vi "PH_IEEE1394Camera.get further Cam Information.vi"(0 "i ref in":refnum<vi>, 2 "IMAQ1394 Session In":T1, 4 "Cam Error in":errorcluster, 5 "error in (no error)":errorcluster) -> (14 "i ref out":refnum<vi>, 16 "IMAQ1394 Session Out":T1, 18 "Cam Error out":errorcluster, 19 "error out":errorcluster)   [LabVIEW 2014, in "PH_IEEE1394Camera.lvlib"]
doc: "This VI gets the cam model and wrties it to own attributes and GUI element."
uses:
  PH_IEEE1394Camera.lvlib
  <vilib>/userdefined/High Color/IMAQdx.ctl
  <resource>/objmgr/imaqdx.rc
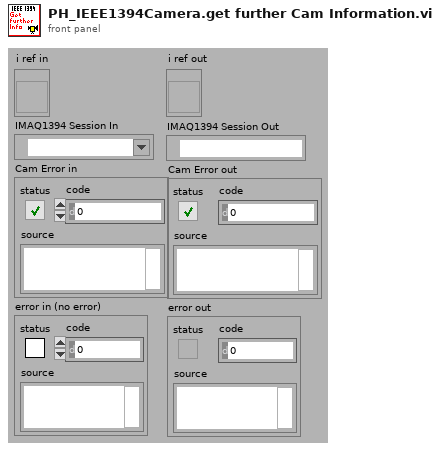
[diagram p1: front panel]
types:
  T1 = typedef "IMAQdx.ctl" = refnum<k21>
  T2 = typedef "PH_IEEE1394Camera.lvlib/PH_IEEE1394Camera.i attribute.ctl" = cluster{"Gui Refs":cluster{"Brightness":refnum<vi>, "Shutter":refnum<vi>, "Gain":refnum<vi>, "Center of Gravity":refnum<vi>, "Supported Video Modes":refnum<vi>, "Trigger Polarity":refnum<vi>, "Trigger Mode":refnum<vi>, "Trigger Timeout":refnum<vi>, "Bit Depth":refnum<vi>, "Video Mode":refnum<vi>, "Top":refnum<vi>, "Bottom":refnum<vi>, "Left":refnum<vi>, "Right":refnum<vi>, "Set ROI to Maximum":refnum<vi>, "Camera Details":refnum<vi>, "Current Cam Attributes":refnum<vi>, "Attribute to set":refnum<vi>, "Num Value":refnum<vi>, "String Value":refnum<vi>, "Bool Value":refnum<vi>, "Set Cam Attribute":refnum<vi>}, "Cam":cluster{"IMAQ1394 Session":T1, "Camera Details":T3}, "Current Attributes":T4[], "Supported Video Modes ":cluster{"Video Mode":u32, "Video Mode Name":string}[], "Wanted Attributes":cluster{"Name":string, "Num Value":dbl, "String Value":string, "Boolean Value":bool}[], "Cam Attributes":T6}
  T3 = typedef "PH_IEEE1394Camera.lvlib/PH_IEEE1394Camera.Cam Details.ctl" = cluster{"Model":string, "Serial Number":dbl, "Cam name (Machinery)":string, "Bus Type":string}
  T4 = typedef "PH_IEEE1394Camera.lvlib/PH_IEEE1394Camera.Cam Attribute.ctl" = cluster{"Information":cluster{"Type":T5, "Readable":bool, "Writable":bool, "Name":string}, "Num Value":dbl, "String Value":string, "Maximum":dbl, "Minimum":dbl, "Units":string, "Description":string, "EnumStrings[]":string[], "EnumValues[]":u32[], "Boolean Value":bool}
  T5 = typedef "NI_Vision_Acquisition_Software.lvlib/IMAQdx Attribute Type.ctl" = enum32{"U32", "I64", "DBL", "String", "Enum", "Bool", "Command"}
  T6 = typedef "PH_IEEE1394Camera.lvlib/PH_IEEE1394Camera.Relevant Cam Attributes.ctl" = cluster{"Video Mode":cluster{"Name":string, "Index":i32}, "Brightness":cluster{"Name":string, "Index":i32}, "Gain":cluster{"Name":string, "Index":i32}, "Shutter":cluster{"Name":string, "Index":i32}, "Trigger Pol":cluster{"Name":string, "Index":i32}, "Trigger Mode":cluster{"Name":string, "Index":i32}, "Timeout":cluster{"Name":string, "Index":i32}, "Bit Depth":cluster{"Name":string, "Index":i32}, "Pixel Bits":cluster{"Name":string, "Index":i32}, "Pixel Bytes":cluster{"Name":string, "Index":i32}, "Left":cluster{"Name":string, "Index":i32}, "Right":cluster{"Name":string, "Index":i32}, "Top":cluster{"Name":string, "Index":i32}, "Bottom":cluster{"Name":string, "Index":i32}}
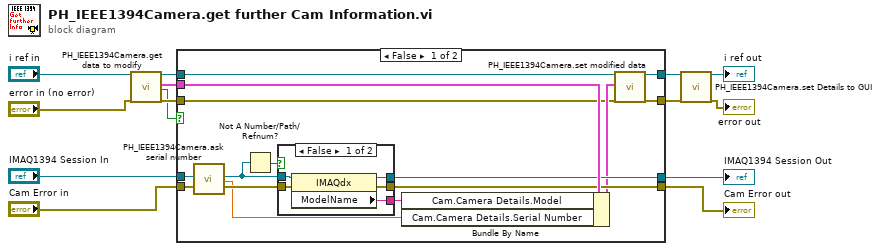
[diagram p0: block diagram]
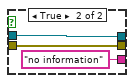
[diagram p2: hidden frame]
diagram:
  n1 = call "PH_IEEE1394Camera.get data to modify.vi"("i ref in"="i ref in", "error in (no error)"="error in (no error)") -> ("i ref out"=w11:refnum<vi>, "i attribute"=w7:T2, "timed out"=w6:bool, "error out"=w12:errorcluster)  [unwired: 14 in]
  n2 = case shown="False" w6 {
    tunnel: [w22 w39] -> w14
    tunnel: w12 -> [w15 w40]
    tunnel: w11 -> [w29 w41]
    tunnel: [w28 w40] -> w10
    tunnel: [w27 w41] -> w3
    tunnel: "IMAQ1394 Session In" -> [w21 w39]
    tunnel: w7 -> [w24 _]
    tunnel: "Cam Error in" -> [w19 w38]
    tunnel: [w23 w38] -> w4
    frame False {
      n3 = call "PH_IEEE1394Camera.ask serial number.vi"("IMAQ1394 Session In"=w21, "Cam Error in"=w19) -> ("IMAQ1394 Session Out"=w20:T1, "Serial Number"=w17:dbl, "Cam Error out"=w18:errorcluster)  [unwired: 15 in]
      n4 = Not A Number/Path/Refnum?(number/path/refnum=w20) -> (NaN/Path/Refnum?=w26:bool)
      n5 = case shown="False" w26 {
        tunnel: w20 -> [w34 w37]
        tunnel: [w32 w37] -> w22
        tunnel: w18 -> [w33 w36]
        tunnel: [w30 "no information"] -> w25
        tunnel: [w31 w36] -> w23
        frame False {
          n6 = property class="IMAQdx"(reference=w34, error in=w33) -> (reference out=w32:T1, error out=w31:errorcluster, "ModelName"=w30:string)
        }
        frame True {
        }
      }
      n7 = Bundle By Name(cluster=w24, "Cam.Camera Details.Model"=w25, "Cam.Camera Details.Serial Number"=w17) -> (w16:T2)
      n8 = call "PH_IEEE1394Camera.set modified data.vi"("i ref in"=w29, "i attribute"=w16, "error in (no error)"=w15) -> ("i ref out"=w27:refnum<vi>, "error out"=w28:errorcluster)  [unwired: 15 in]
    }
    frame True {
    }
  }
  "IMAQ1394 Session Out" <- w14
  "Cam Error out" <- w4
  n9 = call "PH_IEEE1394Camera.set Details to GUI.vi"("VI in"=w3, "error in (no error)"=w10) -> ("VI out"=→"i ref out":refnum<vi>, "error out"=→"error out":errorcluster)  [unwired: 16 in]
